vi "Cluster - Unbundle.vi"() -> ()   [LabVIEW 2016]
panel:
  out "Boolean":bool
  out "String":string
  out "Numeric":dbl
  in  "Cluster":T1
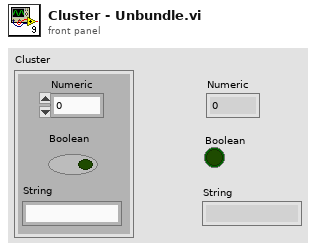
[diagram p1: front panel]
types:
  T1 = cluster{"Numeric":dbl, "Boolean":bool, "String":string}
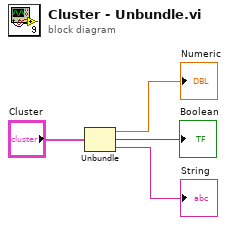
[diagram p0: block diagram]
diagram:
  n1 = Unbundle("Cluster") -> ("Numeric"=→"Numeric":dbl, "Boolean"=→"Boolean":bool, "String"=→"String":string)
